vi "Write.vi"(10 "U32":u32, 11 "U32 in":refnum<class "U32.lvclass">) -> (3 "U32 out":refnum<class "U32.lvclass">)   [LabVIEW 2020, in "Data.lvlib" / "U32.lvclass"]
doc: "Write U32."
uses:
  U32.lvclass
  U32.lvclass/U32.ctl
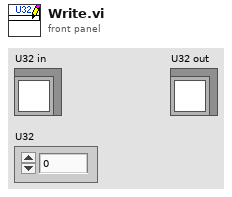
[diagram p1: front panel]
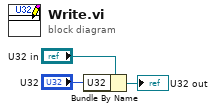
[diagram p0: block diagram]
diagram:
  n1 = Bundle By Name(cluster="U32 in", "U32"="U32") -> (→"U32 out":refnum<class "U32.lvclass">)
